vi "Read task.vi"(8 "error in (no error)":errorcluster, 11 "NI_DAQmx(Angular) in":refnum<class "NI_DAQmx(Angular).lvclass">) -> (0 "error out":errorcluster, 2 "task":refnum<k21>, 3 "NI_DAQmx(Angular) out":refnum<class "NI_DAQmx(Angular).lvclass">)   [LabVIEW 2025, in "NI_DAQmx(Angular).lvclass"]
uses:
  NI_DAQmx(Angular).lvclass
  NI_DAQmx(Angular).lvclass/NI_DAQmx(Angular).ctl
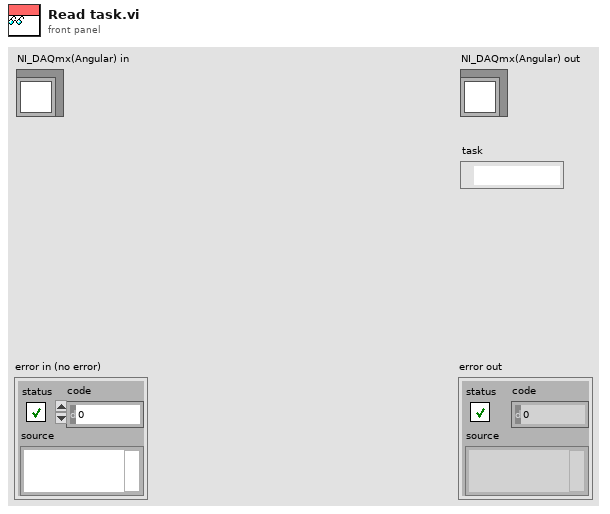
[diagram p1: front panel]
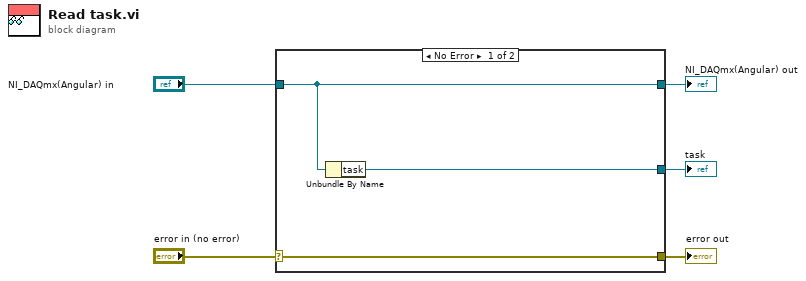
[diagram p0: block diagram]
diagram:
  n1 = case shown="No Error" "error in (no error)" {
    selector: "error in (no error)" -> [w8 w9]
    tunnel: [w8 w9] -> w4
    tunnel: [w7 w10] -> w2
    tunnel: "NI_DAQmx(Angular) in" -> [w7 w10]
    tunnel: [w6 _] -> w1
    frame No Error {
      n2 = Unbundle By Name(w7) -> ("task"=w6:refnum<k21>)
    }
    frame Error {
    }
  }
  "error out" <- w4
  "NI_DAQmx(Angular) out" <- w2
  "task" <- w1
